vi "TLB Native Dynamic Events ver 0.04f.vi"() -> ()   [LabVIEW 2018]
uses:
  Labview Training Phase 2/Enum Controls/States for Action Engine.ctl
  Type def/TLB event states.ctl
  Type def/TLB MHL States.ctl
  <vilib>/Studica/Studica Toolkit/Background/I2C Channel.ctl
  <vilib>/Studica/Studica Toolkit/NavX/NavX.lvlib
  <vilib>/myRIO/Common/Instrument Driver Framework/myRIO v1.0/AI/typedefs/AI Channels Enum.ctl
  <vilib>/myRIO/Common/Instrument Driver Framework/myRIO v1.0/AI/typedefs/AI Channels List.ctl
  <vilib>/Studica/Studica Toolkit/Background/Mxp Selection.ctl
  <vilib>/ptbypt/NI_PtbyPt.lvlib
panel:
  out "NavX Info Out":T2
  out "LinearAcceleration":T3
  out "Displacement":T4
  out "YRPHfH":T5
  in  "y":dbl=-1.2 format="%#_13g"
  out "Distance":T6
  in  "Return to IDLE":bool
  out "Sharp IR Distance":dbl
  out "Sharp IR Distance 2":dbl
  out "CM":fxp<+,64,16>
  out "Ultrasonic sensor":dbl format="%0.2f"
  out "Waveform Chart 3":dbl(graph)
  in  "xTargetSpeed":dbl
  in  "yTargetSpeed":dbl
  in  "wTargetSpeed":dbl
  out "Speed":T7
  in  "Reset Encoder 0":bool
  out "Action Queue Items":i32
  out "State Logic Queue Items":i32
  out "Action Queues items":string[](array[string])=["Hardware reset", "Software reset", ""]
  out "State logic":T8=enum."Task 2"
  out "Action State":string
  in  "Tasks Selector":string(combo)="Task 2"
  in  "Stop Queue":bool
  in  "Start Task":bool
  # "Test Programme written by Calvin Loke    Dated: 28 Aug 2019\nTest Programme revised by Dr Alex See   Dated 30 Aug 2019\n\nProgramme version:   TLB Native Dynamic Events ver 0.04b.vi"
  # "System Health Status Update"
  # "Sequence of Actions"
  # "Continuous (Repeated)"
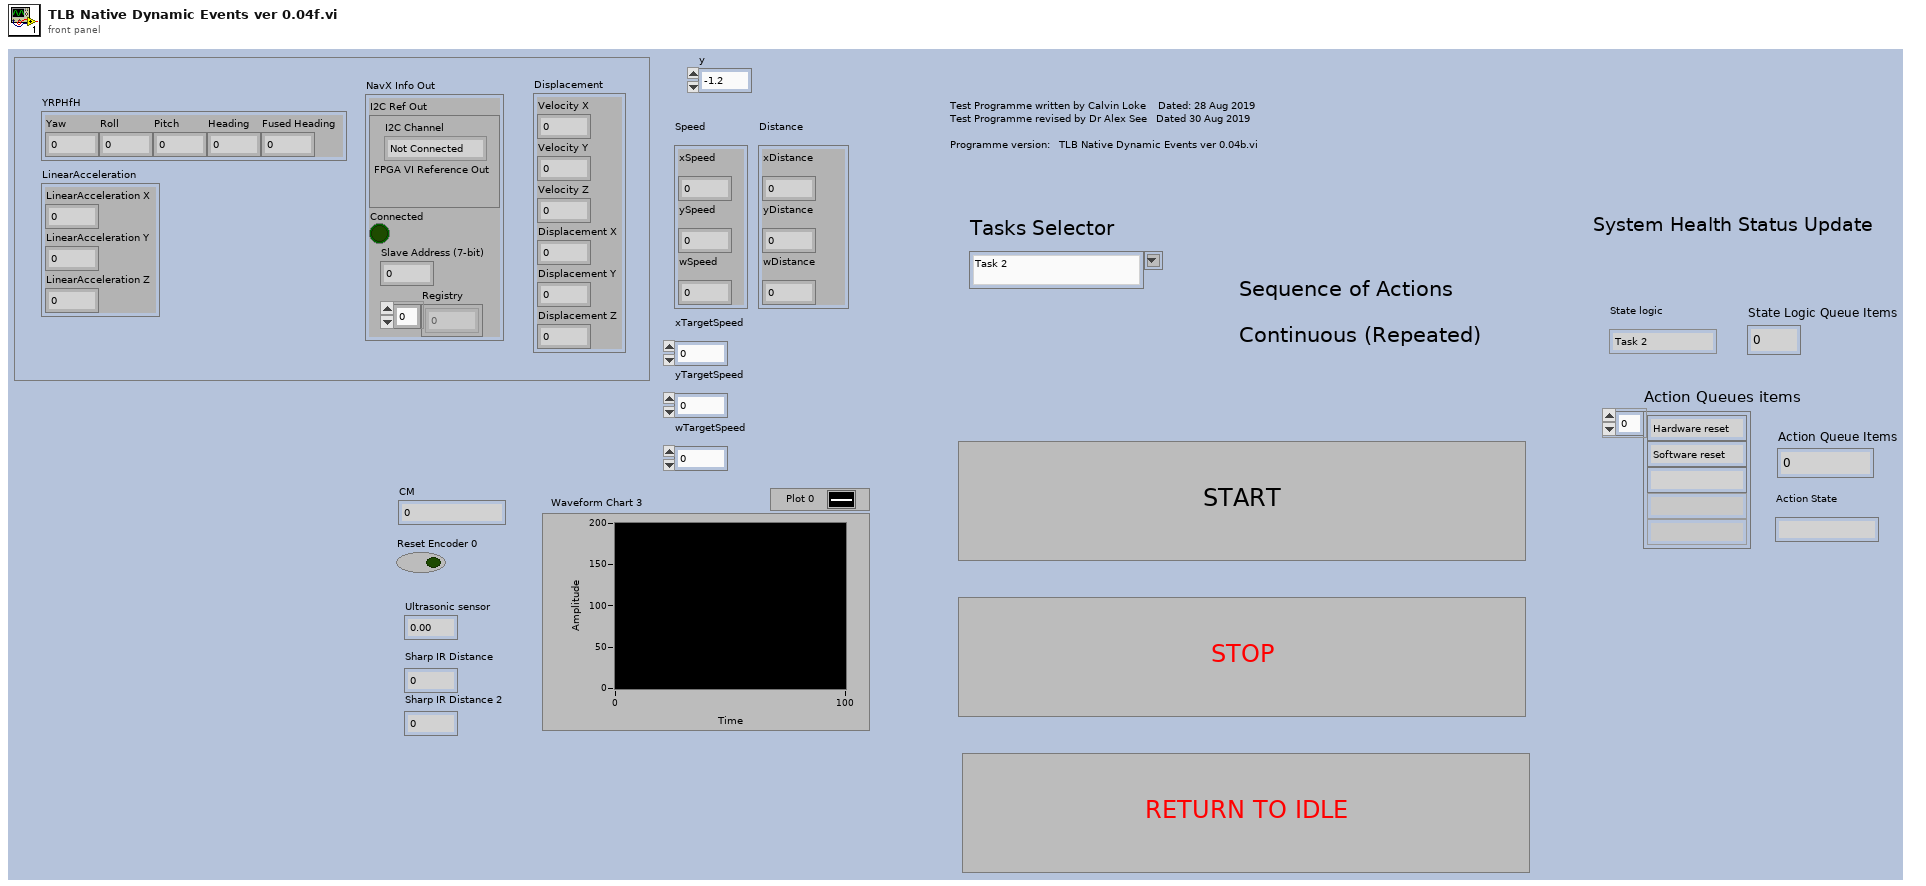
[diagram p1: front panel]
types:
  T1 = typedef "I2C Channel.ctl" = enum16{"Not Connected", "A", "B"}
  T2 = cluster{"I2C Ref Out":cluster{"I2C Channel":T1, "FPGA VI Reference Out":refnum<k20>}, "Connected":bool, "Slave Address (7-bit)":u8, "Registry":u8[]}
  T3 = cluster{"LinearAcceleration X":dbl, "LinearAcceleration Y":dbl, "LinearAcceleration Z":dbl}
  T4 = cluster{"Velocity X":dbl, "Velocity Y":dbl, "Velocity Z":dbl, "Displacement X":dbl, "Displacement Y":dbl, "Displacement Z":dbl}
  T5 = cluster{"Yaw":dbl, "Roll":dbl, "Pitch":dbl, "Heading":dbl, "Fused Heading":dbl}
  T6 = cluster{"xDistance":dbl, "yDistance":dbl, "wDistance":dbl}
  T7 = cluster{"xSpeed":dbl, "ySpeed":dbl, "wSpeed":dbl}
  T8 = typedef "TLB MHL States.ctl" = enum16{"None", "Startup", "Idle", "Processing", "Shutdown", "Reset", "Task 1", "Task 2", "Task 3", "Task 4", "Task 4a", "Task 4b", "Task 4c", "Task 4d", "Task 4e", "Task 4f", "Task 4g", "Task 4h", "Acquire image", "Wall follow mode", "Autodrive", "Autodrive a"}
  T9 = typedef "States for Action Engine.ctl" = enum16{"Initialize", "Write", "Read"}
  T10 = typedef "TLB event states.ctl" = enum16{"Start Sequence", "Exit", "Start Task 1", "Start Task 2", "Start Task 3", "Start Task 4", "Camera vision", "Wall follow mode", "Idle", "Start Drive Straight"}
  T11 = typedef "Mxp Selection.ctl" = enum16{"MXP A", "MXP B"}
  T12 = typedef "AI Channels List.ctl" = T13[]
  T13 = typedef "AI Channels Enum.ctl" = enum16{"Not Connected", "AudioIn/Left", "AudioIn/Right", "C/AI0", "C/AI1", "A/AI0", "A/AI1", "A/AI2", "A/AI3", "A/AI4", "A/AI5", "A/AI6", "A/AI7", "B/AI0", "B/AI1", "B/AI2", "B/AI3", "B/AI4", "B/AI5", "B/AI6", "B/AI7", "AI/AI0", "AI/AI1", "AI/AI2", "AI/AI3", "A/AI0 (DIFF)", "A/AI1 (DIFF)", "A/AI2 (DIFF)", "A/AI3 (DIFF)", "B/AI0 (DIFF)", "B/AI1 (DIFF)", "B/AI2 (DIFF)", "B/AI3 (DIFF)"}
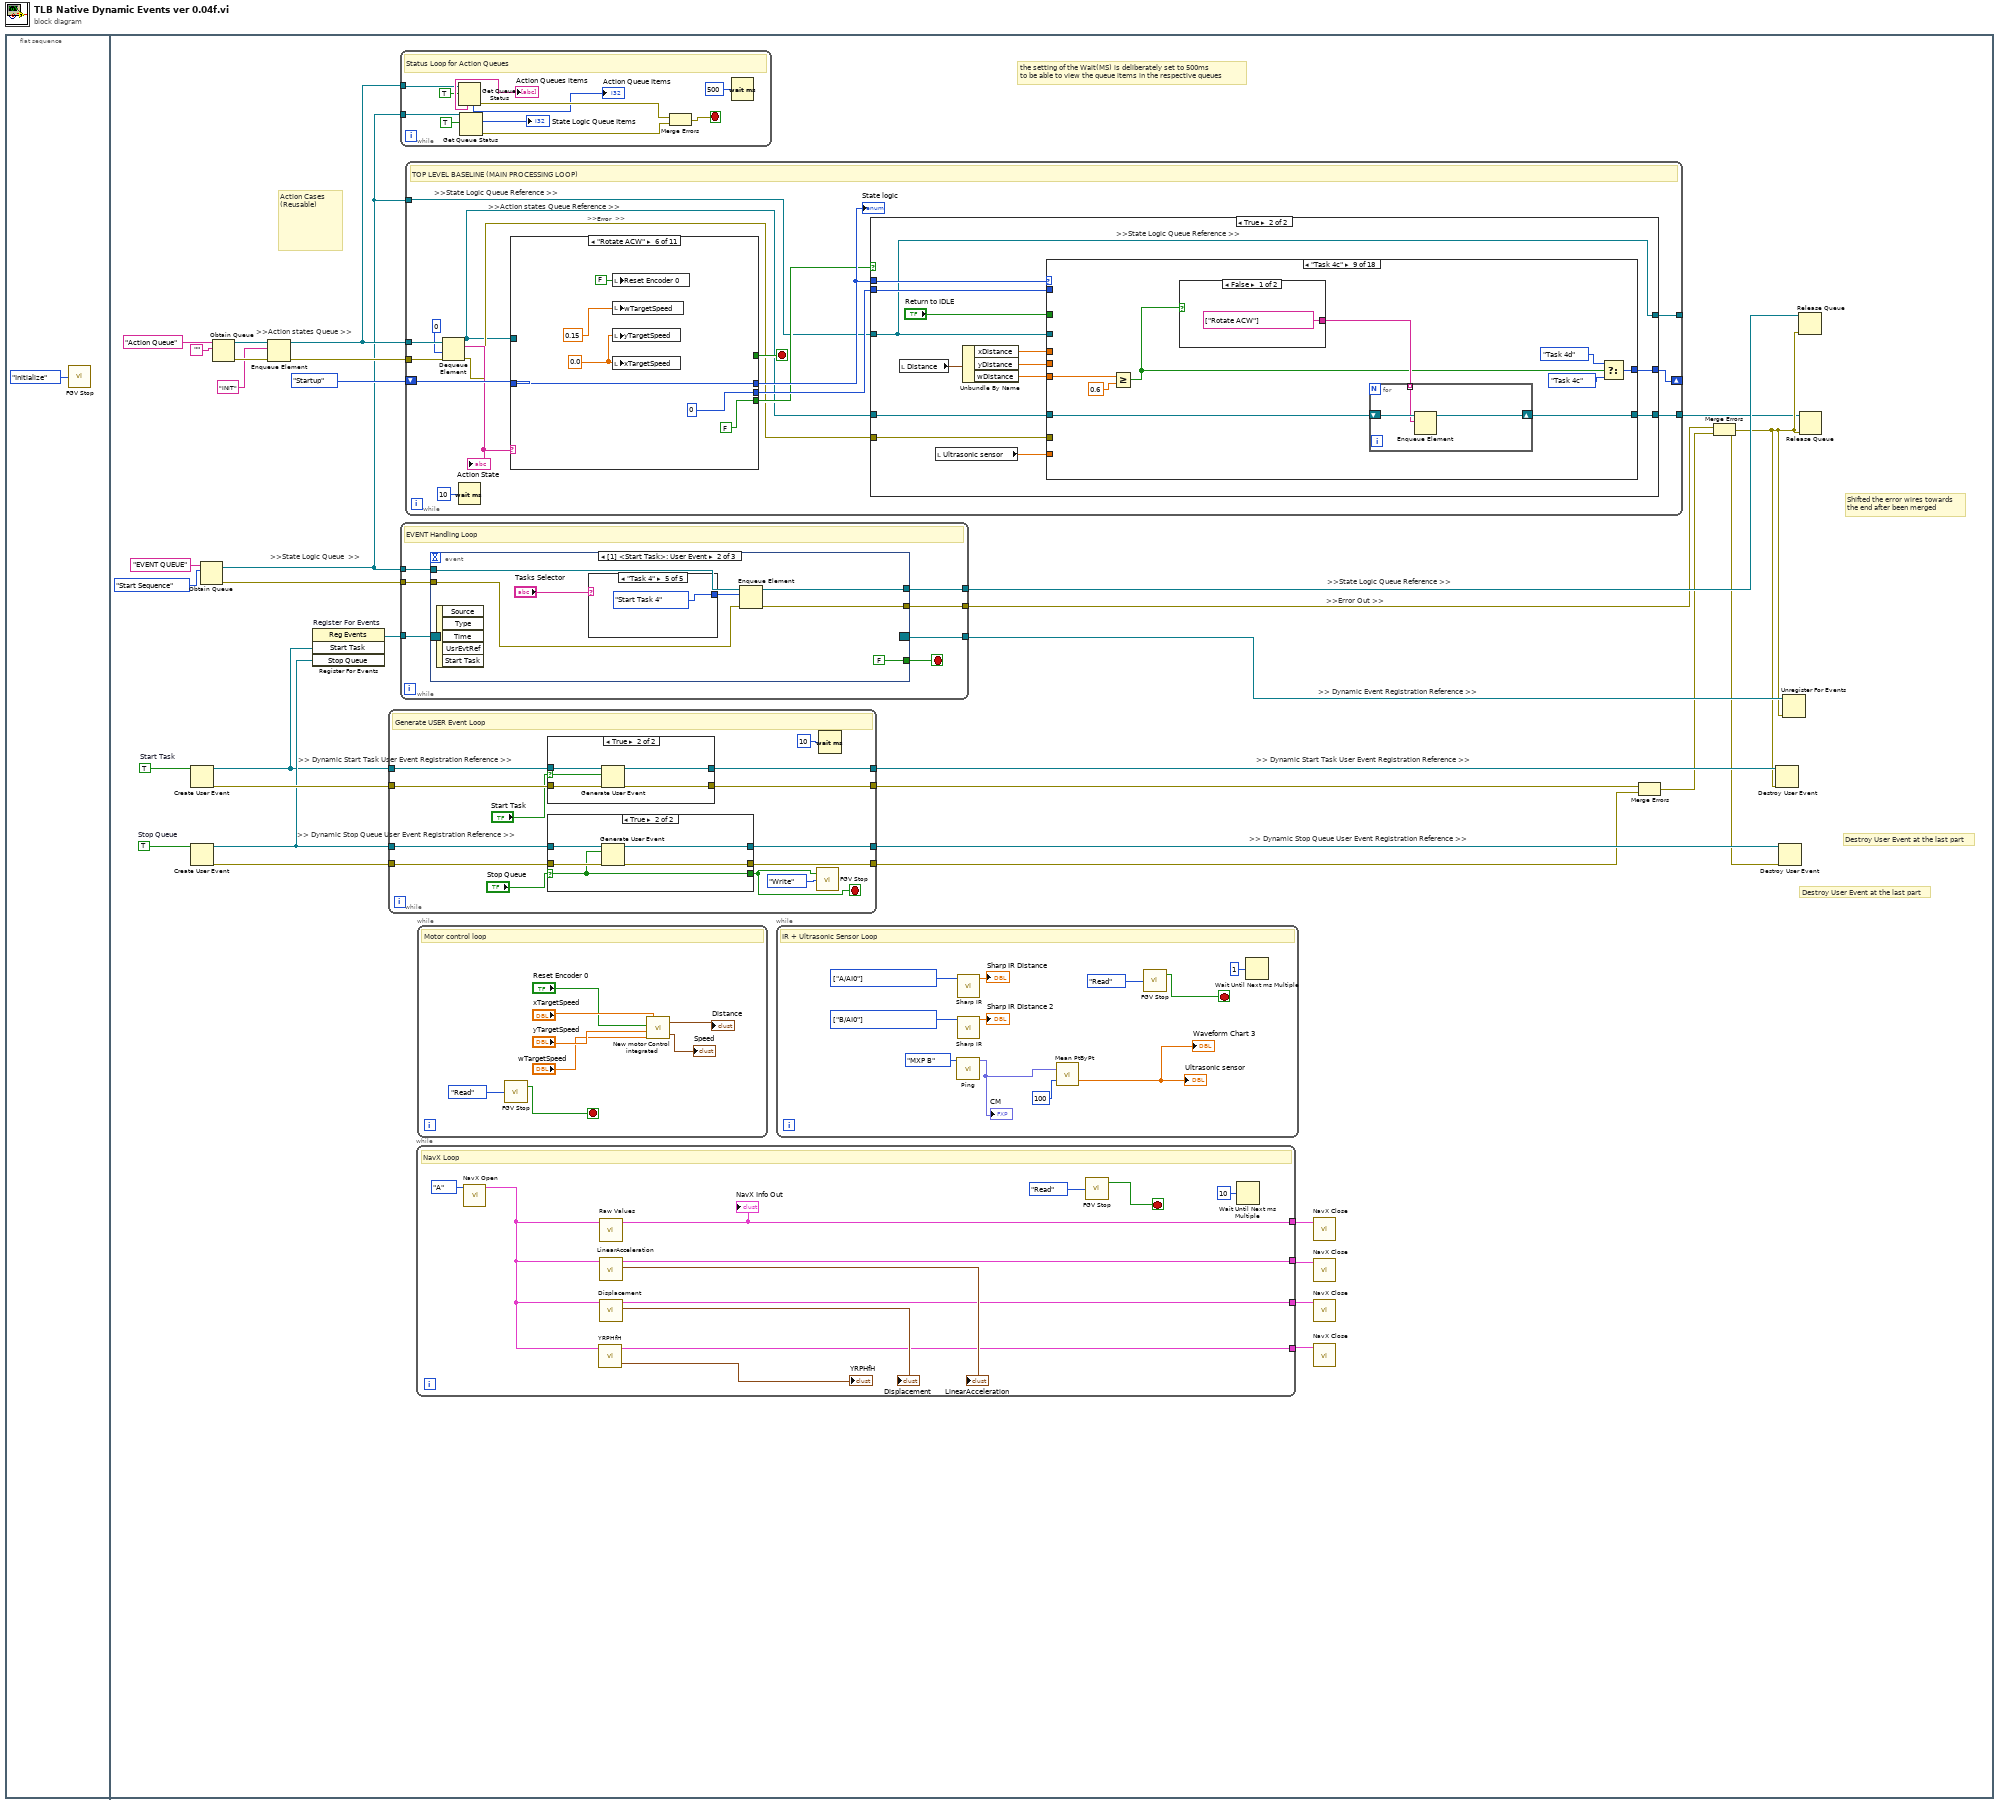
[diagram p0: block diagram]
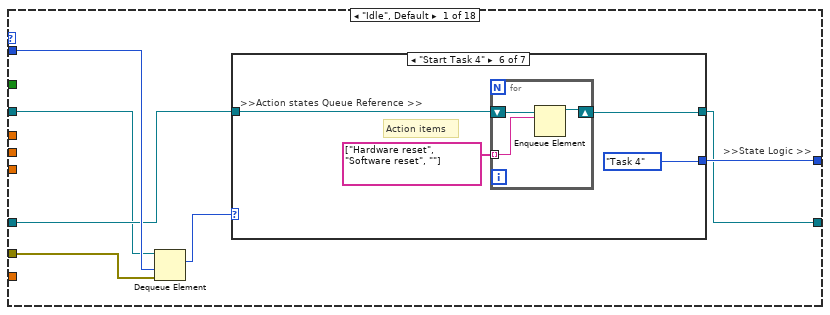
[diagram p3: hidden frame]
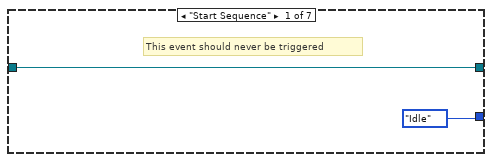
[diagram p4: hidden frame]
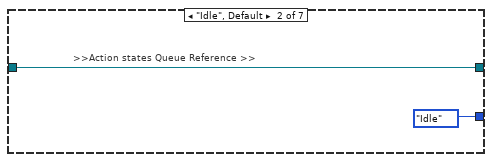
[diagram p5: hidden frame]
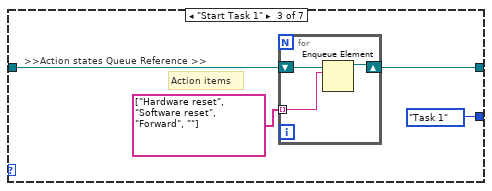
[diagram p6: hidden frame]
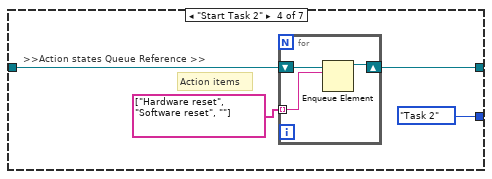
[diagram p7: hidden frame]
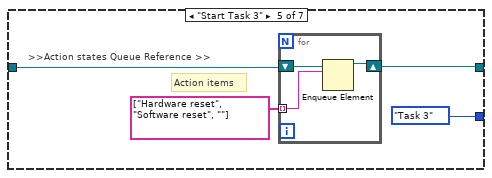
[diagram p8: hidden frame]
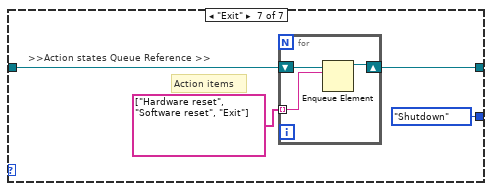
[diagram p9: hidden frame]
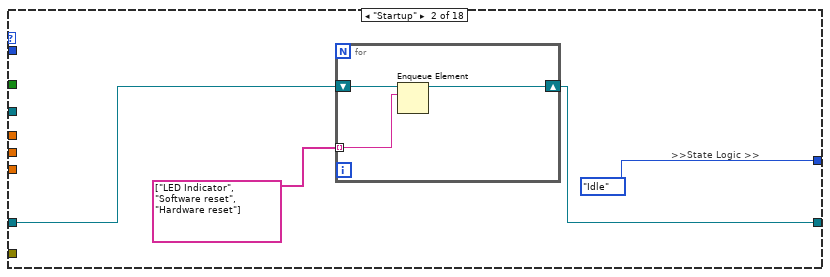
[diagram p10: hidden frame]
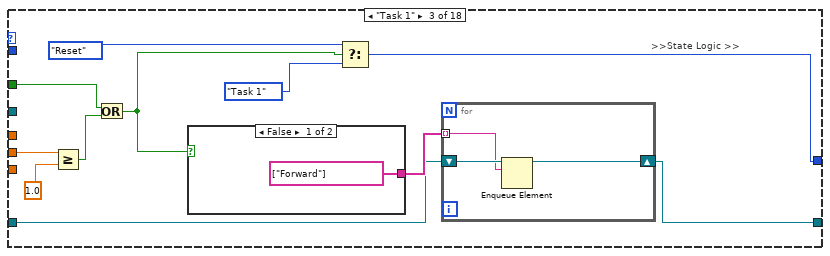
[diagram p11: hidden frame]
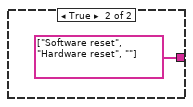
[diagram p12: hidden frame]
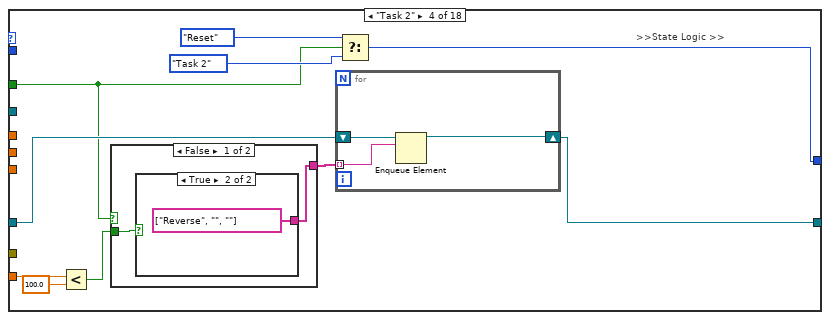
[diagram p13: hidden frame]
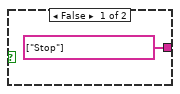
[diagram p14: hidden frame]
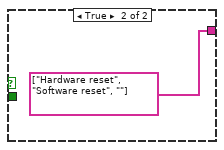
[diagram p15: hidden frame]
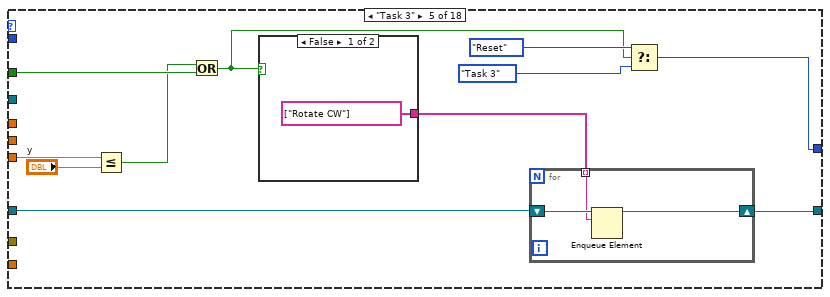
[diagram p16: hidden frame]
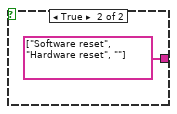
[diagram p17: hidden frame]
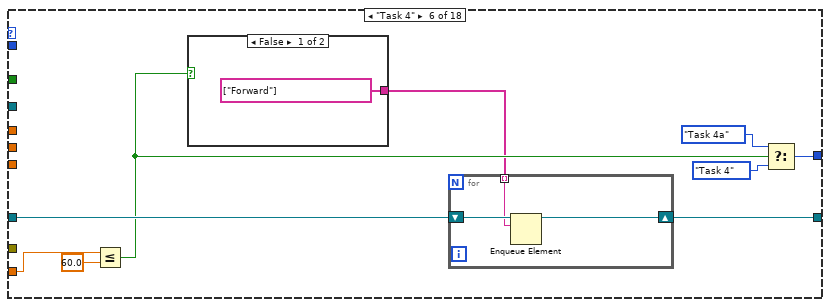
[diagram p18: hidden frame]
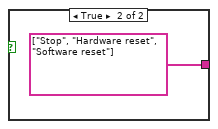
[diagram p19: hidden frame]
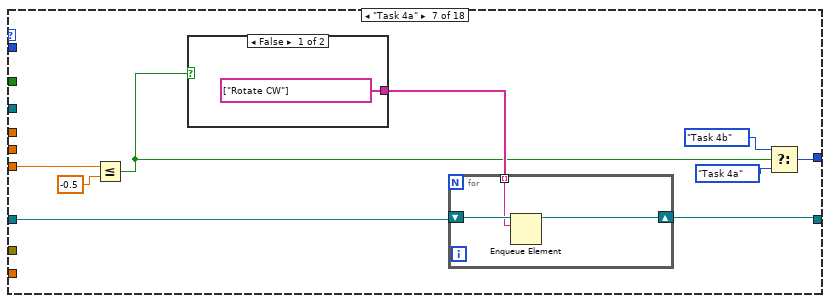
[diagram p20: hidden frame]
diagram:
  n1 = flat-sequence {
    frame #0 {
      n2 = call "FGV Stop.vi"("Init/Read/Write State"=States_for_Action_Engine."Initialize") -> ()  [unwired: 2 in, 2 out]
    }
    frame #1 {
      w34 = TRUE  # Stop Queue
      w33 = TRUE  # Start Task
      # "the setting of the Wait(MS) is deliberately set to 500ms\nto be able to view the queue items in the respective queues"
      # "Action Cases\n(Reusable)"
      # ">>Error Out >>"
      # ">> Dynamic Stop Queue User Event Registration Reference >>"
      # ">> Dynamic Start Task User Event Registration Reference >>"
      # ">> Dynamic Stop Queue User Event Registration Reference >>"
      # ">> Dynamic Start Task User Event Registration Reference >>"
      # ">> Dynamic Event Registration Reference >>"
      # ">>Action states Queue >>"
      # ">>State Logic Queue  >>"
      # ">>State Logic Queue Reference >>"
      # "Destroy User Event at the last part"
      # "Destroy User Event at the last part"
      # "Shifted the error wires towards\nthe end after been merged"
      n3 = Create User Event(user event datatype=w33) -> (user event=w25:refnum<user-event>, error out=w30:errorcluster)  [unwired: 1 in]
      n4 = Create User Event(user event datatype=w34) -> (user event=w26:refnum<user-event>, error out=w29:errorcluster)  [unwired: 1 in]
      n5 = Obtain Queue(name (unnamed)="EVENT QUEUE", element data type=TLB_event_states."Start Sequence" ("Enum")) -> (queue out=w9:refnum<queue>, error out=w15:errorcluster)  [unwired: 3 in, 1 out]
      n6 = Obtain Queue(name (unnamed)="Action Queue", element data type="") -> (queue out=w18:refnum<queue>, error out=w14:errorcluster)  [unwired: 3 in, 1 out]
      n7 = Enqueue Element(queue=w18, element="INIT", error in (no error)=w14) -> (queue out=w10:refnum<queue>, error out=w13:errorcluster)  [unwired: 1 in, 1 out]
      n8 = register-events "Register For Events"(w25, w26) -> (reference out=w24:refnum<event-registration>)  [unwired: 2 in, 1 out]
      n9 = while {
        tunnel: w25 -> [w451]
        tunnel: w26 -> [w450]
        tunnel: [w449] -> w32
        tunnel: [w448] -> w31
        tunnel: w30 -> [w447]
        tunnel: [w446] -> w28
        tunnel: w29 -> [w445]
        tunnel: [w444] -> w27
        stop <- w440 stop-if-true
        # "Generate USER Event Loop"
        n10 = case shown="True" "Start Task" {
          selector: "Start Task" -> [_ w463]
          tunnel: w451 -> [w462 w467]
          tunnel: [w462 w466] -> w448
          tunnel: w447 -> [w461 w465]
          tunnel: [w461 w464] -> w446
          frame False {
          }
          frame True {
            n11 = Generate User Event(user event=w467, event data cluster=w463, error in=w465) -> (user event out=w466:refnum<user-event>, error out=w464:errorcluster)  [unwired: 1 in]
          }
        }
        n12 = case shown="True" "Stop Queue" {
          selector: "Stop Queue" -> [_ w456]
          tunnel: w450 -> [w455 w460]
          tunnel: [w455 w459] -> w449
          tunnel: w445 -> [w454 w458]
          tunnel: [w454 w457] -> w444
          tunnel: [FALSE w456] -> w440
          frame False {
          }
          frame True {
            n13 = Generate User Event(user event=w460, event data cluster=w456, error in=w458) -> (user event out=w459:refnum<user-event>, error out=w457:errorcluster)  [unwired: 1 in]
          }
        }
        n14 = call "FGV Stop.vi"("Init/Read/Write State"=States_for_Action_Engine."Write", "Input Node"=w440) -> ()  [unwired: 1 in, 2 out]
        n15 = Wait (ms)(milliseconds to wait=u32 10) -> ()  [unwired: 1 out]
      }
      n16 = while {
        tunnel: w10 -> [w74]
        tunnel: w9 -> [w71]
        stop <- w68 stop-if-true
        # "Status Loop for Action Queues"
        n17 = Get Queue Status(queue=w74, return elements? (F)=TRUE) -> (error out=w70:errorcluster, # elements in queue=→"Action Queue Items":i32, elements=→"Action Queues items":string[])  [unwired: 1 in, 5 out]
        n18 = Get Queue Status(queue=w71, return elements? (F)=TRUE) -> (# pending remove=→"State Logic Queue Items":i32, error out=w69:errorcluster)  [unwired: 1 in, 6 out]
        n19 = Merge Errors(w70, w69) -> (w68:errorcluster)
        n20 = Wait (ms)(milliseconds to wait=u32 500) -> ()  [unwired: 1 out]
      }
      n21 = while {
        tunnel: w24 -> [w415]
        tunnel: [w414] -> w23
        tunnel: w9 -> [w412]
        tunnel: [w411] -> w22
        tunnel: w15 -> [w410]
        tunnel: [w409] -> w12
        stop <- w413 stop-if-true
        # "EVENT Handling Loop"
        n22 = event shown="[1] <Start Task>: User Event" {
          selector: w415 -> [_ _ _]
          dyn-events: [_ _ _] -> w414
          timeout: _ -> [_ _ _]
          tunnel: [FALSE FALSE w439] -> w413
          tunnel: w412 -> [w420 w427 w437]
          tunnel: [w419 w426 w438] -> w411
          tunnel: w410 -> [w417 w423 w435]
          tunnel: [w416 w422 w434] -> w409
          event Timeout {
            n23 = event-data() -> ()  [unwired: 1 in, 3 out]
            n24 = Enqueue Element(queue=w420, element=TLB_event_states."Idle" ("Enum"), error in (no error)=w417) -> (queue out=w419:refnum<queue>, error out=w416:errorcluster)  [unwired: 1 in, 1 out]
          }
          event User Event {
            n25 = event-data() -> ()  [unwired: 1 in, 5 out]
            n26 = case shown="\"Task 4\"" "Tasks Selector" {
              tunnel: [TLB_event_states."Idle" ("Enum") TLB_event_states."Start Task 1" ("Enum") TLB_event_states."Start Task 2" ("Enum") TLB_event_states."Start Task 3" ("Enum") TLB_event_states."Start Task 4" ("Enum")] -> w424
              frame Default {
              }
              frame "Task 1" {
              }
              frame "Task 2" {
              }
              frame "Task 3" {
              }
              frame "Task 4" {
              }
            }
            n27 = Enqueue Element(queue=w427, element=w424, error in (no error)=w423) -> (queue out=w426:refnum<queue>, error out=w422:errorcluster)  [unwired: 1 in, 1 out]
          }
          event User Event {
            n28 = event-data() -> ("Stop Queue"=w439:bool)  [unwired: 1 in, 4 out]
            n29 = Enqueue Element At Opposite End(queue=w437, element=TLB_event_states."Exit" ("Enum"), error in (no error)=w435) -> (queue out=w438:refnum<queue>, error out=w434:errorcluster)  [unwired: 1 in, 1 out]
          }
        }
      }
      n30 = while {
        tunnel: w9 -> [w79]
        shift-right: [w84] -> _
        shift-left: TLB_MHL_States."Startup" ("Enum") -> [w91]
        tunnel: w10 -> [w89]
        tunnel: w13 -> [w87]
        tunnel: [w86] -> _
        tunnel: [w85] -> w7
        stop <- w82 stop-if-true
        # ">>Error  >>"
        # ">>Action states Queue Reference >>"
        # ">>State Logic Queue Reference >>"
        # "TOP LEVEL BASELINE (MAIN PROCESSING LOOP)"
        n31 = Dequeue Element(queue=w89, timeout in ms (-1)=0, error in (no error)=w87) -> (queue out=w77:refnum<queue>, element=w88:string, error out=w78:errorcluster)  [unwired: 1 out]
        "Action State" <- w88
        n32 = Wait (ms)(milliseconds to wait=u32 10) -> ()  [unwired: 1 out]
        n33 = case shown="\"Rotate ACW\"" w88 {
          tunnel: [w359 w364 w367 w372 w377 w385 w390 w395 w399 w404 TLB_MHL_States."Shutdown" ("Enum")] -> w90
          tunnel: w91 -> [w359 w364 w367 w372 w377 w385 w390 w395 w399 w404 _]
          tunnel: [w358 0 0 0 0 0 0 0 0 0 0] -> w83
          tunnel: [_ _ _ _ _ _ _ _ _ _ TRUE] -> w82
          tunnel: [TRUE FALSE FALSE FALSE FALSE FALSE FALSE FALSE FALSE FALSE FALSE] -> w81
          tunnel: w77 -> [_ _ _ _ _ _ _ _ _ _ _]
          frame "No action", Default {
            n34 = case shown="\"Idle\"" w359 {
              tunnel: [0 100] -> w358
              frame "Startup", Default {
              }
              frame "Idle" {
              }
            }
          }
          frame "Init" {
            # ">>State Logic  >>"
          }
          frame "LED Indicator" {
          }
          frame "Forward" {
            w368 = 0.0
            n35 = local write "Reset Encoder 0"(FALSE ("Reset Encoder 0")) -> ()
            n36 = local write "wTargetSpeed"(w368) -> ()
            n37 = local write "yTargetSpeed"(0.5 ("yTargetSpeed")) -> ()
            n38 = local write "xTargetSpeed"(w368) -> ()
          }
          frame "Rotate CW" {
            w374 = 0.0
            n39 = local write "Reset Encoder 0"(FALSE ("Reset Encoder 0")) -> ()
            n40 = local write "wTargetSpeed"(-0.15 ("yTargetSpeed")) -> ()
            n41 = local write "yTargetSpeed"(w374) -> ()
            n42 = local write "xTargetSpeed"(w374) -> ()
          }
          frame "Rotate ACW" {
            w382 = 0.0
            n43 = local write "Reset Encoder 0"(FALSE ("Reset Encoder 0")) -> ()
            n44 = local write "wTargetSpeed"(0.15 ("yTargetSpeed")) -> ()
            n45 = local write "yTargetSpeed"(w382) -> ()
            n46 = local write "xTargetSpeed"(w382) -> ()
          }
          frame "Reverse" {
            w386 = 0.0
            n47 = local write "Reset Encoder 0"(FALSE ("Reset Encoder 0")) -> ()
            n48 = local write "wTargetSpeed"(w386) -> ()
            n49 = local write "yTargetSpeed"(-0.3 ("yTargetSpeed")) -> ()
            n50 = local write "xTargetSpeed"(w386) -> ()
          }
          frame "Stop" {
            w392 = 0.0
            n51 = local write "Reset Encoder 0"(FALSE ("Reset Encoder 0")) -> ()
            n52 = local write "wTargetSpeed"(w392) -> ()
            n53 = local write "yTargetSpeed"(w392) -> ()
            n54 = local write "xTargetSpeed"(w392) -> ()
          }
          frame "Software reset" {
          }
          frame "Hardware reset" {
            w400 = 0.0
            n55 = local write "Reset Encoder 0"(TRUE ("Reset Encoder 0")) -> ()
            n56 = local write "wTargetSpeed"(w400) -> ()
            n57 = local write "yTargetSpeed"(w400) -> ()
            n58 = local write "xTargetSpeed"(w400) -> ()
          }
          frame "Exit" {
          }
        }
        "State logic" <- w90
        n59 = case shown="True" w81 {
          tunnel: w90 -> [w94 w108]
          tunnel: w79 -> [w95 w102]
          tunnel: w77 -> [w93 w107]
          tunnel: [w95 w102] -> w86
          tunnel: [w93 w106] -> w85
          tunnel: [w94 w105] -> w84
          tunnel: w78 -> [_ w104]
          tunnel: w83 -> [_ w103]
          frame False {
          }
          frame True {
            # ">>State Logic Queue Reference >>"
            n60 = local read "Distance"() -> (w100:T6)
            n61 = local read "Ultrasonic sensor"() -> (w98:dbl)
            n62 = Unbundle By Name(w100) -> ("xDistance"=w96:dbl, "yDistance"=w99:dbl, "wDistance"=w97:dbl)
            n63 = case shown="\"Task 4c\"" w108 {
              tunnel: w102 -> [w109 _ _ _ _ _ _ _ _ _ _ _ _ _ _ _ _ _]
              tunnel: w107 -> [w111 w156 w168 w183 w205 w216 w227 w243 w256 w270 w285 w299 w312 w327 w340 w346 w349 w355]
              tunnel: [w110 w155 w167 w184 w204 w217 w226 w242 w254 w269 w284 w298 w313 w326 w339 w346 w348 w355] -> w106
              tunnel: [w114 TLB_MHL_States."Idle" ("Enum") w170 w185 w201 w220 w232 w241 w257 w268 w282 w297 w310 w325 TLB_MHL_States."Idle" ("Enum") TLB_MHL_States."Reset" ("Enum") TLB_MHL_States."Shutdown" ("Enum") TLB_MHL_States."Reset" ("Enum")] -> w105
              tunnel: w104 -> [w112 _ _ _ _ _ _ _ _ _ _ _ _ _ _ _ _ _]
              tunnel: w103 -> [w113 _ _ _ _ _ _ _ _ _ _ _ _ _ _ _ _ _]
              tunnel: "Return to IDLE" -> [_ _ w165 w180 w199 _ _ _ _ _ _ _ _ _ _ _ _ _]
              tunnel: w99 -> [_ _ w164 _ _ _ _ w240 _ w271 _ w296 _ w324 _ _ _ _]
              tunnel: w98 -> [_ _ _ w182 _ w215 _ _ _ _ _ _ _ _ _ _ _ _]
              tunnel: w97 -> [_ _ _ _ w198 _ w229 _ w255 _ w283 _ w311 _ _ _ _ _]
              tunnel: w96 -> [_ _ _ _ _ _ _ _ _ _ _ _ _ _ _ _ _ _]
              frame "Idle", Default {
                # ">>State Logic >>"
                n64 = Dequeue Element(queue=w109, timeout in ms (-1)=w113, error in (no error)=w112) -> (element=w115:T10)  [unwired: 3 out]
                n65 = case shown="\"Start Task 4\"" w115 {
                  tunnel: [TLB_MHL_States."Idle" ("Enum") TLB_MHL_States."Idle" ("Enum") TLB_MHL_States."Task 1" ("Enum") TLB_MHL_States."Task 2" ("Enum") TLB_MHL_States."Task 3" ("Enum") TLB_MHL_States."Task 4" ("Enum") TLB_MHL_States."Shutdown" ("Enum")] -> w114
                  tunnel: [w117 w118 w122 w127 w136 w142 w148] -> w110
                  tunnel: w111 -> [w117 w118 w120 w128 w137 w143 w149]
                  frame "Start Sequence" {
                    # "This event should never be triggered"
                  }
                  frame "Idle", Default {
                    # ">>Action states Queue Reference >>"
                  }
                  frame "Start Task 1" {
                    # ">>Action states Queue Reference >>"
                    # "Action items"
                    n66 = for {
                      shift-right: [w126] -> w122
                      shift-left: w120 -> [w125]
                      tunnel: string[] ["Hardware reset", "Software reset", "Forward", ""] -> [w124] mode=indexing
                      n67 = Enqueue Element(queue=w125, element=w124) -> (queue out=w126:refnum<queue>)  [unwired: 2 in, 2 out]
                    }
                  }
                  frame "Start Task 2" {
                    # ">>Action states Queue Reference >>"
                    # "Action items"
                    n68 = for {
                      shift-right: [w133] -> w127
                      shift-left: w128 -> [w132]
                      tunnel: string[] ["Hardware reset", "Software reset", ""] -> [w131] mode=indexing
                      n69 = Enqueue Element(queue=w132, element=w131) -> (queue out=w133:refnum<queue>)  [unwired: 2 in, 2 out]
                    }
                  }
                  frame "Start Task 3" {
                    # ">>Action states Queue Reference >>"
                    # "Action items"
                    n70 = for {
                      shift-right: [w140] -> w136
                      shift-left: w137 -> [w139]
                      tunnel: string[] ["Hardware reset", "Software reset", ""] -> [w138] mode=indexing
                      n71 = Enqueue Element(queue=w139, element=w138) -> (queue out=w140:refnum<queue>)  [unwired: 2 in, 2 out]
                    }
                  }
                  frame "Start Task 4" {
                    # ">>Action states Queue Reference >>"
                    # "Action items"
                    n72 = for {
                      shift-right: [w147] -> w142
                      shift-left: w143 -> [w146]
                      tunnel: string[] ["Hardware reset", "Software reset", ""] -> [w145] mode=indexing
                      n73 = Enqueue Element(queue=w146, element=w145) -> (queue out=w147:refnum<queue>)  [unwired: 2 in, 2 out]
                    }
                  }
                  frame "Exit" {
                    # ">>Action states Queue Reference >>"
                    # "Action items"
                    n74 = for {
                      shift-right: [w154] -> w148
                      shift-left: w149 -> [w153]
                      tunnel: string[] ["Hardware reset", "Software reset", "Exit"] -> [w152] mode=indexing
                      n75 = Enqueue Element(queue=w153, element=w152) -> (queue out=w154:refnum<queue>)  [unwired: 2 in, 2 out]
                    }
                  }
                }
              }
              frame "Startup" {
                # ">>State Logic >>"
                n76 = for {
                  shift-right: [w160] -> w155
                  shift-left: w156 -> [w161]
                  tunnel: string[] ["LED Indicator", "Software reset", "Hardware reset"] -> [w159] mode=indexing
                  n77 = Enqueue Element(queue=w161, element=w159) -> (queue out=w160:refnum<queue>)  [unwired: 2 in, 2 out]
                }
              }
              frame "Task 1" {
                # ">>State Logic >>"
                n78 = Greater Or Equal?(x=w164, y=1.0) -> (x >= y?=w162:bool)
                n79 = Or(x=w165, y=w162) -> (x .or. y?=w166:bool)
                n80 = case shown="False" w166 {
                  tunnel: [string[] ["Forward"] string[] ["Software reset", "Hardware reset", ""]] -> w169
                  frame False {
                  }
                  frame True {
                  }
                }
                n81 = Select(t=TLB_MHL_States."Reset" ("Enum"), s=w166, f=TLB_MHL_States."Task 1" ("Enum")) -> (s? t:f=w170:T8)
                n82 = for {
                  shift-right: [w176] -> w167
                  shift-left: w168 -> [w177]
                  tunnel: w169 -> [w175] mode=indexing
                  n83 = Enqueue Element(queue=w177, element=w175) -> (queue out=w176:refnum<queue>)  [unwired: 2 in, 2 out]
                }
              }
              frame "Task 2" {
                # ">>State Logic >>"
                n84 = Less?(x=w182, y=100.0) -> (x < y?=w178:bool)
                n85 = case shown="False" w180 {
                  tunnel: [w188 string[] ["Hardware reset", "Software reset", ""]] -> w179
                  tunnel: w178 -> [w189 _]
                  frame False {
                    n86 = case shown="True" w189 {
                      tunnel: [string[] ["Stop"] string[] ["Reverse", "", ""]] -> w188
                      frame False {
                      }
                      frame True {
                      }
                    }
                  }
                  frame True {
                  }
                }
                n87 = for {
                  shift-right: [w194] -> w184
                  shift-left: w183 -> [w195]
                  tunnel: w179 -> [w193] mode=indexing
                  n88 = Enqueue Element(queue=w195, element=w193) -> (queue out=w194:refnum<queue>)  [unwired: 2 in, 2 out]
                }
                n89 = Select(t=TLB_MHL_States."Reset" ("Enum"), s=w180, f=TLB_MHL_States."Task 2" ("Enum")) -> (s? t:f=w185:T8)
              }
              frame "Task 3" {
                n90 = Less Or Equal?(x=w198, y="y") -> (x <= y?=w196:bool)
                n91 = Or(x=w196, y=w199) -> (x .or. y?=w200:bool)
                n92 = case shown="False" w200 {
                  tunnel: [string[] ["Rotate CW"] string[] ["Software reset", "Hardware reset", ""]] -> w206
                  frame False {
                  }
                  frame True {
                  }
                }
                n93 = for {
                  shift-right: [w208] -> w204
                  shift-left: w205 -> [w209]
                  tunnel: w206 -> [w207] mode=indexing
                  n94 = Enqueue Element(queue=w209, element=w207) -> (queue out=w208:refnum<queue>)  [unwired: 2 in, 2 out]
                }
                n95 = Select(t=TLB_MHL_States."Reset" ("Enum"), s=w200, f=TLB_MHL_States."Task 3" ("Enum")) -> (s? t:f=w201:T8)
              }
              frame "Task 4" {
                n96 = Less Or Equal?(x=w215, y=60.0) -> (x <= y?=w213:bool)
                n97 = case shown="False" w213 {
                  tunnel: [string[] ["Forward"] string[] ["Stop", "Hardware reset", "Software reset"]] -> w212
                  frame False {
                  }
                  frame True {
                  }
                }
                n98 = for {
                  shift-right: [w224] -> w217
                  shift-left: w216 -> [w225]
                  tunnel: w212 -> [w223] mode=indexing
                  n99 = Enqueue Element(queue=w225, element=w223) -> (queue out=w224:refnum<queue>)  [unwired: 2 in, 2 out]
                }
                n100 = Select(t=TLB_MHL_States."Task 4a" ("Enum"), s=w213, f=TLB_MHL_States."Task 4" ("Enum")) -> (s? t:f=w220:T8)
              }
              frame "Task 4a" {
                n101 = Less Or Equal?(x=w229, y=-0.5) -> (x <= y?=w228:bool)
                n102 = case shown="False" w228 {
                  tunnel: [string[] ["Rotate CW"] string[] ["Stop", "Hardware reset", "Software reset"]] -> w230
                  frame False {
                  }
                  frame True {
                  }
                }
                n103 = for {
                  shift-right: [w238] -> w226
                  shift-left: w227 -> [w239]
                  tunnel: w230 -> [w237] mode=indexing
                  n104 = Enqueue Element(queue=w239, element=w237) -> (queue out=w238:refnum<queue>)  [unwired: 2 in, 2 out]
                }
                n105 = Select(t=TLB_MHL_States."Task 4b" ("Enum"), s=w228, f=TLB_MHL_States."Task 4a" ("Enum")) -> (s? t:f=w232:T8)
              }
              frame "Task 4b" {
                n106 = Greater Or Equal?(x=w240, y=0.15) -> (x >= y?=w244:bool)
                n107 = case shown="False" w244 {
                  tunnel: [string[] ["Forward"] string[] ["Stop", "Hardware reset", "Software reset"]] -> w245
                  frame False {
                  }
                  frame True {
                  }
                }
                n108 = for {
                  shift-right: [w252] -> w242
                  shift-left: w243 -> [w253]
                  tunnel: w245 -> [w251] mode=indexing
                  n109 = Enqueue Element(queue=w253, element=w251) -> (queue out=w252:refnum<queue>)  [unwired: 2 in, 2 out]
                }
                n110 = Select(t=TLB_MHL_States."Task 4c" ("Enum"), s=w244, f=TLB_MHL_States."Task 4b" ("Enum")) -> (s? t:f=w241:T8)
              }
              frame "Task 4c" {
                n111 = Greater Or Equal?(x=w255, y=0.6) -> (x >= y?=w258:bool)
                n112 = case shown="False" w258 {
                  tunnel: [string[] ["Rotate ACW"] string[] ["Stop", "Hardware reset", "Software reset"]] -> w259
                  frame False {
                  }
                  frame True {
                  }
                }
                n113 = for {
                  shift-right: [w266] -> w254
                  shift-left: w256 -> [w267]
                  tunnel: w259 -> [w265] mode=indexing
                  n114 = Enqueue Element(queue=w267, element=w265) -> (queue out=w266:refnum<queue>)  [unwired: 2 in, 2 out]
                }
                n115 = Select(t=TLB_MHL_States."Task 4d" ("Enum"), s=w258, f=TLB_MHL_States."Task 4c" ("Enum")) -> (s? t:f=w257:T8)
              }
              frame "Task 4d" {
                n116 = Greater Or Equal?(x=w271, y=0.6) -> (x >= y?=w272:bool)
                n117 = case shown="False" w272 {
                  tunnel: [string[] ["Forward"] string[] ["Stop", "Hardware reset", "Software reset"]] -> w273
                  frame False {
                  }
                  frame True {
                  }
                }
                n118 = for {
                  shift-right: [w280] -> w269
                  shift-left: w270 -> [w281]
                  tunnel: w273 -> [w279] mode=indexing
                  n119 = Enqueue Element(queue=w281, element=w279) -> (queue out=w280:refnum<queue>)  [unwired: 2 in, 2 out]
                }
                n120 = Select(t=TLB_MHL_States."Task 4e" ("Enum"), s=w272, f=TLB_MHL_States."Task 4d" ("Enum")) -> (s? t:f=w268:T8)
              }
              frame "Task 4e" {
                n121 = Greater Or Equal?(x=w283, y=0.6) -> (x >= y?=w286:bool)
                n122 = case shown="False" w286 {
                  tunnel: [string[] ["Rotate ACW"] string[] ["Stop", "Hardware reset", "Software reset"]] -> w287
                  frame False {
                  }
                  frame True {
                  }
                }
                n123 = for {
                  shift-right: [w294] -> w284
                  shift-left: w285 -> [w295]
                  tunnel: w287 -> [w293] mode=indexing
                  n124 = Enqueue Element(queue=w295, element=w293) -> (queue out=w294:refnum<queue>)  [unwired: 2 in, 2 out]
                }
                n125 = Select(t=TLB_MHL_States."Task 4f" ("Enum"), s=w286, f=TLB_MHL_States."Task 4e" ("Enum")) -> (s? t:f=w282:T8)
              }
              frame "Task 4f" {
                n126 = Greater Or Equal?(x=w296, y=0.6) -> (x >= y?=w300:bool)
                n127 = case shown="False" w300 {
                  tunnel: [string[] ["Forward"] string[] ["Stop", "Hardware reset", "Software reset"]] -> w301
                  frame False {
                  }
                  frame True {
                  }
                }
                n128 = for {
                  shift-right: [w308] -> w298
                  shift-left: w299 -> [w309]
                  tunnel: w301 -> [w307] mode=indexing
                  n129 = Enqueue Element(queue=w309, element=w307) -> (queue out=w308:refnum<queue>)  [unwired: 2 in, 2 out]
                }
                n130 = Select(t=TLB_MHL_States."Task 4g" ("Enum"), s=w300, f=TLB_MHL_States."Task 4f" ("Enum")) -> (s? t:f=w297:T8)
              }
              frame "Task 4g" {
                n131 = Less Or Equal?(x=w311, y=-0.5) -> (x <= y?=w314:bool)
                n132 = case shown="False" w314 {
                  tunnel: [string[] ["Rotate CW"] string[] ["Stop", "Hardware reset", "Software reset"]] -> w315
                  frame False {
                  }
                  frame True {
                  }
                }
                n133 = for {
                  shift-right: [w322] -> w313
                  shift-left: w312 -> [w323]
                  tunnel: w315 -> [w321] mode=indexing
                  n134 = Enqueue Element(queue=w323, element=w321) -> (queue out=w322:refnum<queue>)  [unwired: 2 in, 2 out]
                }
                n135 = Select(t=TLB_MHL_States."Task 4h" ("Enum"), s=w314, f=TLB_MHL_States."Task 4g" ("Enum")) -> (s? t:f=w310:T8)
              }
              frame "Task 4h" {
                n136 = Greater Or Equal?(x=w324, y=0.6) -> (x >= y?=w328:bool)
                n137 = case shown="False" w328 {
                  tunnel: [string[] ["Forward"] string[] ["Stop", "Hardware reset", "Software reset"]] -> w329
                  frame False {
                  }
                  frame True {
                  }
                }
                n138 = for {
                  shift-right: [w336] -> w326
                  shift-left: w327 -> [w337]
                  tunnel: w329 -> [w335] mode=indexing
                  n139 = Enqueue Element(queue=w337, element=w335) -> (queue out=w336:refnum<queue>)  [unwired: 2 in, 2 out]
                }
                n140 = Select(t=TLB_MHL_States."Idle" ("Enum"), s=w328, f=TLB_MHL_States."Task 4h" ("Enum")) -> (s? t:f=w325:T8)
              }
              frame "Reset" {
                n141 = for {
                  shift-right: [w344] -> w339
                  shift-left: w340 -> [w345]
                  tunnel: string[] ["Software reset", "Hardware reset", ""] -> [w343] mode=indexing
                  n142 = Enqueue Element(queue=w345, element=w343) -> (queue out=w344:refnum<queue>)  [unwired: 2 in, 2 out]
                }
                n143 = Wait (ms)(milliseconds to wait=u32 250) -> ()  [unwired: 1 out]
              }
              frame "Processing" {
              }
              frame "Shutdown" {
                # ">>State Logic >>"
                n144 = for {
                  shift-right: [w353] -> w348
                  shift-left: w349 -> [w354]
                  tunnel: string[] ["Software reset", "Hardware reset", "Exit"] -> [w352] mode=indexing
                  n145 = Enqueue Element(queue=w354, element=w352) -> (queue out=w353:refnum<queue>)  [unwired: 2 in, 2 out]
                }
              }
              frame "None" {
              }
            }
          }
        }
      }
      n146 = while {
        tunnel: [w54] -> w5
        tunnel: [w50] -> w4
        tunnel: [w49] -> w2
        tunnel: [w48] -> w3
        stop <- w56 stop-if-true
        # "NavX Loop"
        n147 = call <vilib>:"NavX Open.vi"("I2C Channel"=I2C_Channel."A") -> ("NavX Info"=w46:T2)  [unwired: 9 in, 1 out]
        n148 = call <vilib>:"YRPHfH.vi"("NavX Info In"=w46) -> ("YRPHfH"=→"YRPHfH":T5, "NavX Info Out"=w49:T2)  [unwired: 3 in]
        n149 = call <vilib>:"Raw Values.vi"("NavX Info In"=w46) -> ("NavX Info Out"=w54:T2)  [unwired: 8 in, 1 out]
        "NavX Info Out" <- w54
        n150 = call <vilib>:"LinearAcceleration.vi"("NavX Info In"=w46) -> ("LinearAcceleration"=→"LinearAcceleration":T3, "NavX Info Out"=w50:T2)  [unwired: 9 in]
        n151 = call <vilib>:"Displacement.vi"("NavX Info In"=w46) -> ("Displacement"=→"Displacement":T4, "NavX Info Out"=w48:T2)  [unwired: 9 in]
        n152 = call "FGV Stop.vi"("Init/Read/Write State"=States_for_Action_Engine."Read") -> ("Output node"=w56:bool)  [unwired: 2 in, 1 out]
        n153 = Wait Until Next ms Multiple(millisecond multiple=u32 10) -> ()  [unwired: 1 out]
      }
      n154 = while {
        stop <- w64 stop-if-true
        # "Motor control loop"
        n155 = call "FGV Stop.vi"("Init/Read/Write State"=States_for_Action_Engine."Read") -> ("Output node"=w64:bool)  [unwired: 2 in, 1 out]
        n156 = call "New motor Control integrated.vi"("wTargetSpeed"="wTargetSpeed", "yTargetSpeed"="yTargetSpeed", "xTargetSpeed"="Reset Encoder 0", "Reset Encoders"="xTargetSpeed") -> ("Speed"=→"Speed":T7, "Distance"=→"Distance":T6)
      }
      n157 = while {
        stop <- w39 stop-if-true
        w44 = T12 [enum."B/AI0"] items=["Not Connected", "AudioIn/Left", "AudioIn/Right", "C/AI0", "C/AI1", "A/AI0", "A/AI1", "A/AI2", "A/AI3", "A/AI4", "A/AI5", "A/AI6", "A/AI7", "B/AI0", "B/AI1", "B/AI2", "B/AI3", "B/AI4", "B/AI5", "B/AI6", "B/AI7", "AI/AI0", "AI/AI1", "AI/AI2", "AI/AI3", "A/AI0 (DIFF)", "A/AI1 (DIFF)", "A/AI2 (DIFF)", "A/AI3 (DIFF)", "B/AI0 (DIFF)", "B/AI1 (DIFF)", "B/AI2 (DIFF)", "B/AI3 (DIFF)"] ("AI Channel")
        w45 = T12 [enum."A/AI0"] items=["Not Connected", "AudioIn/Left", "AudioIn/Right", "C/AI0", "C/AI1", "A/AI0", "A/AI1", "A/AI2", "A/AI3", "A/AI4", "A/AI5", "A/AI6", "A/AI7", "B/AI0", "B/AI1", "B/AI2", "B/AI3", "B/AI4", "B/AI5", "B/AI6", "B/AI7", "AI/AI0", "AI/AI1", "AI/AI2", "AI/AI3", "A/AI0 (DIFF)", "A/AI1 (DIFF)", "A/AI2 (DIFF)", "A/AI3 (DIFF)", "B/AI0 (DIFF)", "B/AI1 (DIFF)", "B/AI2 (DIFF)", "B/AI3 (DIFF)"] ("AI Channel")
        # "IR + Ultrasonic Sensor Loop"
        n158 = call <vilib>:"Ping.vi"("Mxp Side"=Mxp_Selection."MXP B") -> ("CM"=w35:fxp<+,64,16>)  [unwired: 8 in, 2 out]
        "CM" <- w35
        n159 = call <vilib>:"Sharp IR.vi"("AI Channel"=w45) -> ("Sharp IR Distance"=→"Sharp IR Distance":dbl)  [unwired: 8 in, 2 out]
        n160 = call <vilib>:"Sharp IR.vi"("AI Channel"=w44) -> ("Sharp IR Distance"=→"Sharp IR Distance 2":dbl)  [unwired: 8 in, 2 out]
        n161 = call <vilib>:"Mean PtByPt.vi"("x"=w35, "sample length"=100) -> ("mean"=→"Ultrasonic sensor" →"Waveform Chart 3":dbl)  [unwired: 2 in, 1 out]
        n162 = call "FGV Stop.vi"("Init/Read/Write State"=States_for_Action_Engine."Read") -> ("Output node"=w39:bool)  [unwired: 2 in, 1 out]
        n163 = Wait Until Next ms Multiple(millisecond multiple=u32 1) -> ()  [unwired: 1 out]
      }
      n164 = call <vilib>:"NavX Close.vi"("NavX Info In"=w5) -> ()  [unwired: 10 in, 1 out]
      n165 = call <vilib>:"NavX Close.vi"("NavX Info In"=w4) -> ()  [unwired: 10 in, 1 out]
      n166 = call <vilib>:"NavX Close.vi"("NavX Info In"=w3) -> ()  [unwired: 10 in, 1 out]
      n167 = call <vilib>:"NavX Close.vi"("NavX Info In"=w2) -> ()  [unwired: 10 in, 1 out]
      n168 = Merge Errors "Merge Errors"(w28, w27) -> (w6:errorcluster)
      n169 = Merge Errors(w12, w6) -> (w8:errorcluster)
      n170 = Destroy User Event(user event=w31, error in=w8) -> ()  [unwired: 1 out]
      n171 = Destroy User Event(user event=w32, error in=w8) -> ()  [unwired: 1 out]
      n172 = Unregister For Events(event registration refnum=w23, error in=w8) -> ()  [unwired: 1 out]
      n173 = Release Queue(queue=w22, error in (no error)=w8) -> ()  [unwired: 1 in, 3 out]
      n174 = Release Queue(queue=w7, error in (no error)=w8) -> ()  [unwired: 1 in, 3 out]
    }
  }
